vi "Check previous segment window.vi"(9 "Current player segment position":string="75", 10 "Previous player segment position":string="75") -> (2 "Player segment position":string)   [LabVIEW 2013]
uses:
  <vilib>/regexp/Match Regular Expression.xnode
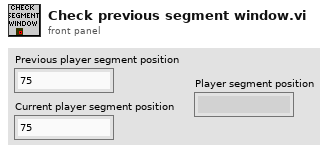
[diagram p1: front panel]
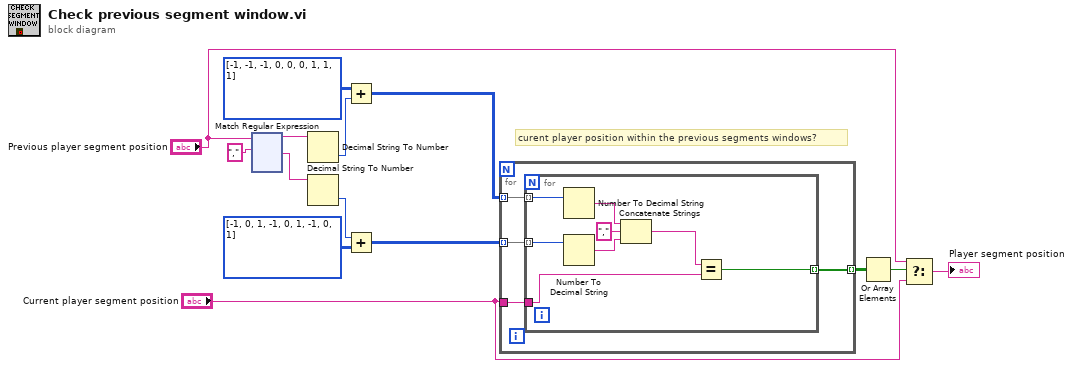
[diagram p0: block diagram]
diagram:
  # "curent player position within the previous segments windows?"
  n1 = xnode "Match Regular Expression"("input string"="Previous player segment position", "regular expression"=",") -> ("before match"=w2:string, "after match"=w1:string)  [unwired: 4 in, 3 out]
  n2 = Decimal String To Number(string=w2) -> (number=w13:i32)  [unwired: 2 in, 1 out]
  n3 = Decimal String To Number(string=w1) -> (number=w12:i32)  [unwired: 2 in, 1 out]
  n4 = Add(x=i32[][] [[-1, -1, -1], [0, 0, 0], [1, 1, 1]], y=w13) -> (x+y=w10:i32[][])
  n5 = Add(x=w12, y=i32[][] [[-1, 0, 1], [-1, 0, 1], [-1, 0, 1]]) -> (x+y=w9:i32[][])
  n6 = for {
    tunnel: w10 -> [w18] mode=indexing
    tunnel: w9 -> [w17] mode=indexing
    tunnel: "Current player segment position" -> [w16]
    tunnel: [w15] -> w8 mode=indexing
    n7 = for {
      tunnel: w18 -> [w26] mode=indexing
      tunnel: w17 -> [w25] mode=indexing
      tunnel: w16 -> [w22]
      tunnel: [w21] -> w15 mode=indexing
      n8 = Number To Decimal String(number=w26) -> (decimal integer string=w24:string)  [unwired: 1 in]
      n9 = Number To Decimal String(number=w25) -> (decimal integer string=w20:string)  [unwired: 1 in]
      n10 = Concatenate Strings(w24, "," ("string"), w20) -> (w23:string)
      n11 = Equal?(x=w23, y=w22) -> (x = y?=w21:bool)
    }
  }
  n12 = Or Array Elements(Boolean array=w8) -> (logical OR=w7:bool)
  n13 = Select(t="Previous player segment position", s=w7, f="Current player segment position") -> (s? t:f=→"Player segment position":string)
